vi "SPD.Config Read Test03 HV_Grid.vi"(8 "Error In":errorcluster, 11 "SPD.Stand Ctrl in":T2 {"spdDeviceSession"."hidSPD.Sturtup Values"."HV_bias" format="%#_6p, V"; "spdDeviceSession"."hidSPD.Sturtup Values"."TSet" format="%#_6p, DegC"; "spdDeviceSession"."hidSPD.Controller"."HV_bias" format="%#_6p, V"; "spdDeviceSession"."hidSPD.Controller"."TSet" format="%#_6p, DegC"}) -> (0 "Error Out":errorcluster, 2 "HV_GridParams":T1, 3 "SPD.Stand Ctrl out":T2 {"spdDeviceSession"."hidSPD.Sturtup Values"."HV_bias" format="%#_6p, V"; "spdDeviceSession"."hidSPD.Sturtup Values"."TSet" format="%#_6p, DegC"; "spdDeviceSession"."hidSPD.Controller"."HV_bias" format="%#_6p, V"; "spdDeviceSession"."hidSPD.Controller"."TSet" format="%#_6p, DegC"})   [LabVIEW 2018]
uses:
  typedefs/SPD.Stand Ctrl.ctl
  Instruments/SPD HID Interface/hidSPDLibForLabView/LibVIs/hidSPD Controls/hidSPD Device Session.ctl
  Instruments/SPD HID Interface/hidSPDLibForLabView/LibVIs/hidSPD Controls/hidSPD Controller.ctl
  Instruments/SPD HID Interface/hidSPDLibForLabView/LibVIs/hidSPD Controls/hidSPD SPD Type.ctl
  Instruments/KC705 DevBoard/typedefs/DevB.Session.ctl
  Instruments/KeySight 53230A/typedefs/FreqC.Session.ctl
  Instruments/KeySight 8164B/KeySight 8164B LAN InstrLib/typedefs/KeySight 8164B control.ctl
  Instruments/LeCroy SDA830/typedefs/LeCroy.Session.ctl
  typedefs/SPD.Events.ctl
  SPD.Config File ctrl.ctl
  <vilib>/Utility/config.llb/Config Data RefNum.ctl
  typedefs/SPD.Meas Result.ctl
  typedefs/SPD.Queues.ctl
  typedefs/SPD.Stand state.ctl
  SPD Measurements/MeasGrid/typedefs/SPD.HV_Grid Test Params.ctl
  <vilib>/Utility/config.llb/Read Key (I32).vi
  <vilib>/Utility/config.llb/Read Key (Double).vi
  <vilib>/Utility/config.llb/NI_LVConfig.lvlib
  Instruments/KeySight 8164B/KeySight 8164B LAN InstrLib.lvlib
  Instruments/SPD HID Interface/hidSPDLibForLabView/hidSPDLibForLabView.lvlib
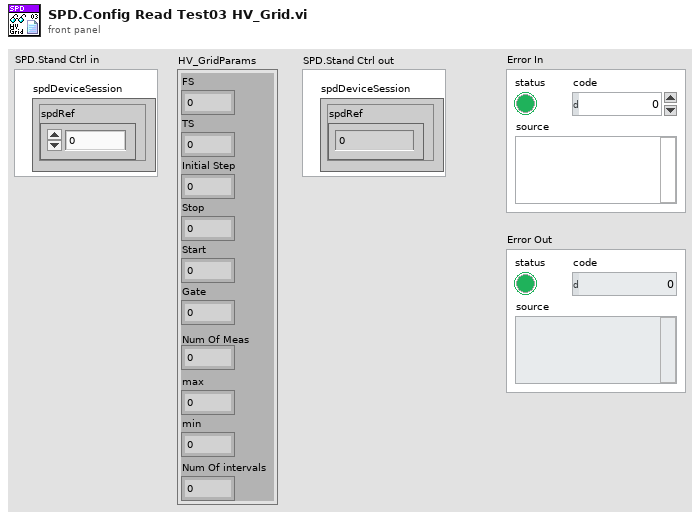
[diagram p1: front panel]
types:
  T1 = typedef "SPD.HV_Grid Test Params.ctl" = cluster{"FS":i32, "TS":i32, "Initial Step":dbl, "Stop":dbl, "Start":dbl, "Gate":dbl, "Num Of Meas":i32, "max":dbl, "min":dbl, "Num Of intervals":i32}
  T2 = typedef "SPD.Stand Ctrl.ctl" = cluster{"spdDeviceSession":T3, "DevBSession":T6, "FreqCSession":T7, "8164BSession":T8, "LeCroySession":T9, "Events":T10, "configFile":T11, "SPD.Result":T13, "SPD.Queues":T14, "Console":refnum<vi>}
  T3 = typedef "hidSPDLibForLabView.lvlib/hidSPD Device Session.ctl" = cluster{"spdRef":u64, "connected":bool, "spdName":string, "hidSPD.Controller":T4, "hidSPD.Sturtup Values":T4, "SPD Type":T5}
  T4 = typedef "hidSPDLibForLabView.lvlib/hidSPD Controller.ctl" = cluster{"TSet":sgl, "HV_bias":sgl, "DDS_stb_code":u16}
  T5 = typedef "hidSPDLibForLabView.lvlib/hidSPD SPD Type.ctl" = enum16{"Free Run", "Strobe"}
  T6 = typedef "DevB.Session.ctl" = cluster{"DevBRef":refnum<visa-resource-name>, "connected":bool}
  T7 = typedef "FreqC.Session.ctl" = cluster{"FreqCRef":refnum<visa-resource-name>, "timeout":dbl, "Gate":dbl, "connected":bool}
  T8 = typedef "KeySight 8164B LAN InstrLib.lvlib/KeySight 8164B control.ctl" = cluster{"Connection ID":refnum<k5>, "Connected":bool, "Info":string, "Slots Info":string[]}
  T9 = typedef "LeCroy.Session.ctl" = cluster{"LeCroySession":refnum<visa-resource-name>, "connected":bool}
  T10 = typedef "SPD.Events.ctl" = cluster{"DCRTest":refnum<user-event>, "Stop":refnum<user-event>}
  T11 = typedef "SPD.Config File ctrl.ctl" = cluster{"configFile ref":T12, "configFile path":path, "equipmentFile ref":T12}
  T12 = typedef "NI_LVConfig.lvlib/Config Data RefNum.ctl" = refnum<k1>
  T13 = typedef "SPD.Meas Result.ctl" = cluster{"HV_Bias":dbl[][][], "Stb_code":dbl[], "Temprature":dbl[], "Data":dbl[][][][], "DateTime":string}
  T14 = typedef "SPD.Queues.ctl" = cluster{"state queue":refnum<queue>}
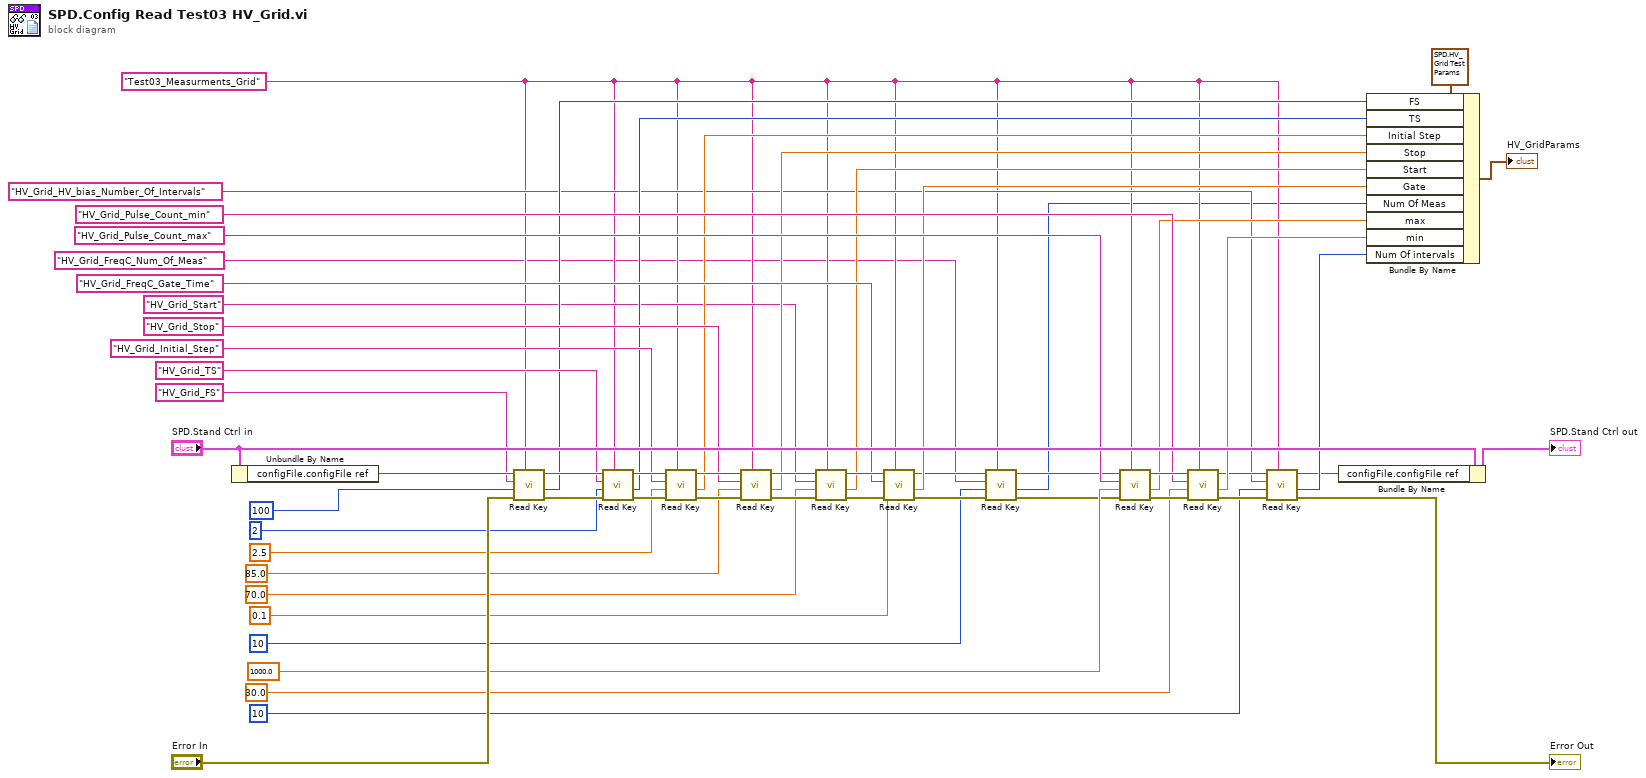
[diagram p0: block diagram]
diagram:
  w7 = "Test03_Measurments_Grid" ("section")
  n1 = Unbundle By Name("SPD.Stand Ctrl in") -> ("configFile.configFile ref"=w55:T12)
  n2 = call-poly <vilib>:"Read Key.vi"("section"=w7, "error in (no error)"="Error In", "default value"=100, "key"="HV_Grid_FS", "refnum"=w55) -> ("error out"=w51:errorcluster, "value"=w26:i32, "refnum out"=w50:T12)  [unwired: 3 in, 1 out]
  n3 = call-poly <vilib>:"Read Key.vi"("section"=w7, "error in (no error)"=w51, "default value"=2, "key"="HV_Grid_TS", "refnum"=w50) -> ("error out"=w46:errorcluster, "value"=w25:i32, "refnum out"=w47:T12)  [unwired: 3 in, 1 out]
  n4 = call-poly <vilib>:"Read Key.vi"("section"=w7, "error in (no error)"=w46, "default value"=2.5, "key"="HV_Grid_Initial_Step", "refnum"=w47) -> ("error out"=w42:errorcluster, "value"=w24:dbl, "refnum out"=w43:T12)  [unwired: 3 in, 1 out]
  n5 = call-poly <vilib>:"Read Key.vi"("section"=w7, "error in (no error)"=w42, "default value"=85.0, "key"="HV_Grid_Stop", "refnum"=w43) -> ("error out"=w38:errorcluster, "value"=w23:dbl, "refnum out"=w39:T12)  [unwired: 3 in, 1 out]
  n6 = call-poly <vilib>:"Read Key.vi"("section"=w7, "error in (no error)"=w38, "default value"=70.0, "key"="HV_Grid_Start", "refnum"=w39) -> ("error out"=w33:errorcluster, "value"=w22:dbl, "refnum out"=w36:T12)  [unwired: 3 in, 1 out]
  n7 = call-poly <vilib>:"Read Key.vi"("section"=w7, "error in (no error)"=w33, "default value"=0.1, "key"="HV_Grid_FreqC_Gate_Time", "refnum"=w36) -> ("error out"=w6:errorcluster, "value"=w21:dbl, "refnum out"=w8:T12)  [unwired: 3 in, 1 out]
  n8 = call-poly <vilib>:"Read Key.vi"("section"=w7, "error in (no error)"=w6, "default value"=10, "key"="HV_Grid_FreqC_Num_Of_Meas", "refnum"=w8) -> ("error out"=w5:errorcluster, "value"=w3:i32, "refnum out"=w4:T12)  [unwired: 3 in, 1 out]
  n9 = call-poly <vilib>:"Read Key.vi"("section"=w7, "error in (no error)"=w5, "default value"=1000.0, "key"="HV_Grid_Pulse_Count_max", "refnum"=w4) -> ("error out"=w31:errorcluster, "value"=w20:dbl, "refnum out"=w32:T12)  [unwired: 3 in, 1 out]
  n10 = call-poly <vilib>:"Read Key.vi"("section"=w7, "error in (no error)"=w31, "default value"=30.0, "key"="HV_Grid_Pulse_Count_min", "refnum"=w32) -> ("error out"=w14:errorcluster, "value"=w19:dbl, "refnum out"=w15:T12)  [unwired: 3 in, 1 out]
  n11 = call-poly <vilib>:"Read Key.vi"("section"=w7, "error in (no error)"=w14, "default value"=10, "key"="HV_Grid_HV_bias_Number_Of_Intervals", "refnum"=w15) -> ("error out"=→"Error Out":errorcluster, "value"=w13:i32, "refnum out"=w12:T12)  [unwired: 3 in, 1 out]
  n12 = Bundle By Name(cluster="SPD.Stand Ctrl in", "configFile.configFile ref"=w12) -> (→"SPD.Stand Ctrl out":T2)
  n13 = Bundle By Name(cluster=T1 {"FS"=0, "TS"=0, "Initial Step"=0.0, "Stop"=0.0, "Start"=0.0, "Gate"=0.0, "Num Of Meas"=0, "max"=0.0, "min"=0.0, "Num Of intervals"=0} ("HV_GridParams"), "FS"=w26, "TS"=w25, "Initial Step"=w24, "Stop"=w23, "Start"=w22, "Gate"=w21, "Num Of Meas"=w3, "max"=w20, "min"=w19, "Num Of intervals"=w13) -> (→"HV_GridParams":T1)
